vi "Custom controls.vi"(0 "Air Ctl":dbl(slide) scale=0.0..10.0, 8 "STOP":bool) -> (4 "Air Indicator":dbl(knob) scale=0.0..10.0, 6 "Waveform Chart":dbl(graph))   [LabVIEW 2020]
doc: "This VI is used for the implementation of custom controls and indicators"
uses:
  Controls/Bool1.ctl
panel:
  out "Boolean":T1
  # "Psi"
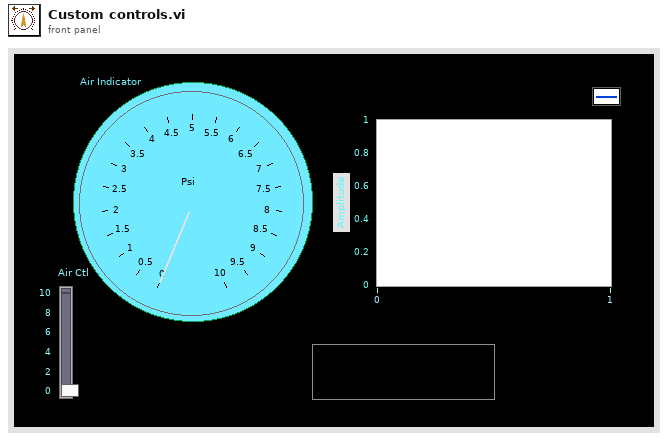
[diagram p1: front panel]
types:
  T1 = typedef "Bool1.ctl" = bool
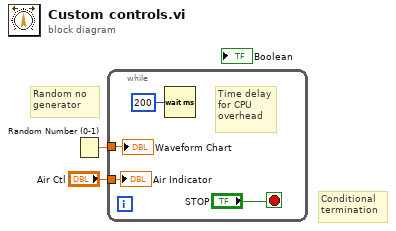
[diagram p0: block diagram]
diagram:
  # "Random no \ngenerator"
  # "Conditional \ntermination"
  n1 = Random Number (0-1)() -> (number: 0 to 1=w2:dbl)
  n2 = while {
    tunnel: w2 -> [w5]
    tunnel: "Air Ctl" -> [w4]
    stop <- "STOP" stop-if-true
    # "Time delay\nfor CPU \noverhead"
    n3 = Wait (ms)(milliseconds to wait=u32 200) -> ()  [unwired: 1 out]
    "Waveform Chart" <- w5
    "Air Indicator" <- w4
  }
